vi "StopEqualization.vi"(8 "error in (no error)":errorcluster, 11 "reference in":refnum<class "niMmWave_Transceiver.lvclass">) -> (0 "error out":errorcluster, 3 "reference out":refnum<class "niMmWave_Transceiver.lvclass">)   [LabVIEW 2019, in "niMmWave_Transceiver.lvclass"]
doc: "Stops calibration procedure"
uses:
  niMmWave_Transceiver.lvclass
  C:/Barkhausen mmWave radar/Development/LV/Barkhausen mmWave hardware control/Host/SubVIs/mmWave instrument_class/mmWave instrument.lvclass
  mmWave instrument_class/Instrument state.ctl
  Low-level/TypeDefs/TX FPGA Reference.ctl
  <vilib>/Utility/error.llb/Error Cluster From Error Code.vi
  <vilib>/rvi/errors/niLvFpgaAdjustHostInterfaceError.vi
  <vilib>/rvi/interface/nirviReadWriteControl/nirviReadWriteControl.xnode
  NiFpgaLv.dll
  <vilib>/rvi/interface/Simulation/niFpgaSimulationCallBeginRW.vi
  mmWave instrument_class/mmWave instrument.lvclass
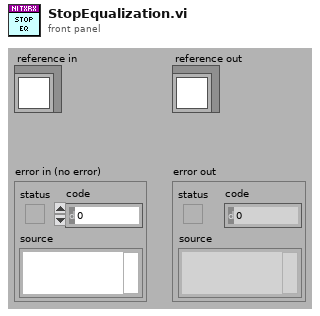
[diagram p1: front panel]
types:
  T1 = typedef "mmWave instrument.lvclass/Instrument state.ctl" = enum16{"Off", "Initialization", "Configuration", "Running", "Calibration"}
  T2 = enum16{"Pass Through", "Tone", "Pulse", "Disable"}
  T3 = typedef "TX FPGA Reference.ctl" = refnum<k20>
  T4 = typedef "niMmWave_Transceiver.lvclass/ObjectAttributesRef.ctl" = refnum<data-value>
  T5 = typedef "niMmWave_Transceiver.lvclass/ObjectAttributes.ctl" = cluster{"session":T6[], "HW.RX resources":T20, "RF config":T21, "RX trigger options":T22, "TX trigger options":T22, "RX samples":i32, "Downloaded Bursts":map{string, T25}, "TX Fs":dbl, "RX Fs":dbl, "burst sequence":string[]}
  T6 = typedef "Session.ctl" = cluster{"3620 session":refnum<queue>, "tx baseband session":T7, "rx baseband session":T15, "tx gain (dB)":dbl, "rx gain (dB)":dbl, "hardware configuration":T16, "gain ranging":T18[], "pxi trigger bus information":T19}
  T7 = typedef "Tx Baseband Session.ctl" = cluster{"3610 session":T8, "7902 reference":T14}
  T8 = typedef "ni3610_and_ni3630_Driver_Lib.lvlib/Main Settings.ctl" = cluster{"VISA resource name":refnum<visa-resource-name>, "Address Space":T9, "window_offset":u32, "register_addresses":T10, "required_MM_fpga_version":cluster{"signature":u32, "hardware":u32, "current revision":u32, "oldest revision":u32}, "CPLD Oldest Compat Version ":cluster{"hardware":u32, "CPLD firmware":u32}, "MM_FPGA_image_location":string, "is_init":bool, "card_type":T11, "DacLmkConfigFileName":string, "AdcLmkConfigFileName":string, "AdcConfigFileName":string, "DacConfigFileName_RevA":string, "DacConfigFileName_RevB":string, "Mulde hardware revision":u8, "bypass DAC PLL\n":bool, "IQ Card Revision":T12, "board capability":T13}
  T9 = typedef "VISA Register Access Address Space.ctl" = u16
  T10 = typedef "ni3610_and_ni3630_Driver_Lib.lvlib/Register Adresses.ctl" = cluster{"MM based Registers":cluster{"Revision":u32, "OldestCompatRev":u32, "signature":u32, "scratch":u32, "LedControl":u32, "BoardHwRev":u32, "BoardControl":u32, "ThermalStatus":u32, "BasebandStatus":u32, "BasebandControl":u32, "BasebandAuxSetup":u32, "BasebandAuxStatus":u32, "LmkSyncOutSetup":u32, " AdcSyncOutSetup":u32, " InjSyncOutSetup":u32, " PxiTrig0OutSetup":u32, " PxiTrig1OutSetup":u32, " PxiTrig2OutSetup":u32, " PxiTrig3OutSetup":u32, " PxiTrig4OutSetup":u32, " PxiTrig5OutSetup":u32, " PxiTrig6OutSetup":u32, " PxiTrig7OutSetup":u32}, "CPLD based Registers":cluster{"SlaveSignature":u32, "SlaveRevision":u32, "SlaveOldestCompatRev":u32, "SlaveScratch":u32, "SlaveSetup":u32, "SlaveStatus":u32, "IDacReg_offset":u32, "LMKRegGrp0_offset":u32, "QDacReg_offset":u32, "BrdTempSensorVal":u32, "TempSensorPowerDown":u32, "GPIOReg_offset":u32, "IAdcReg_offset":u32, "QAdcReg_offset":u32, "LMKRegGrp1_offset":u32, "QadcTempSensorVal":u32, "IadcTempSensorVal":u32, "RevisionReg":u32, "VcxoReg":u32, "CpldStatusReg":u32, "PowerReg":u32, "VBiasEnReg":u32, "ExtRefOeReg":u32, "QdacCtrlReg":u32, "QdacStatusReg":u32, "IdacCtrlReg":u32, "IdacStatusReg":u32, "QdacJtagIn":u32, "QdacJtagOut":u32, "IdacJtagIn":u32, "IdacJtagOut":u32, "IqDcSetupReg":u32, "QadcStatusReg":u32, "IadcStatusReg":u32, "BrdSetupReg":u32, "IqDcRevisionReg":u32, "PllStatusReg":u32, "EndpointScratchReg":u32, "AdcSyncCfgReg":u32, "IqCardOpampReg":u32}, "CPLD Register Offset":u32, "MM  Register Offset":u32, " PxiTrig0OutSetup":u32}
  T11 = typedef "ni3610_and_ni3630_Driver_Lib.lvlib/Base Card Type.ctl" = enum16{"unspecified", "ADC", "DAC"}
  T12 = typedef "ni3610_and_ni3630_Driver_Lib.lvlib/IQ Card Revision.ctl" = enum16{"RevA", "RevB", "RevC", "RevD"}
  T13 = typedef "ni3610_and_ni3630_Driver_Lib.lvlib/Board Capability.ctl" = cluster{"baseband sync":enum16{"no baseband sync", "baseband sync"}}
  T14 = typedef "Blank FPGA Reference.ctl" = refnum<k20>
  T15 = typedef "Rx Baseband Session.ctl" = cluster{"3630 session":T8, "7902 reference":T14}
  T16 = typedef "Hardware Configuration.ctl" = cluster{"direction":T17, "baseband only":bool}
  T17 = typedef "Direction.ctl" = enum16{"Transceiver", "Receiver", "Transmitter"}
  T18 = typedef "Gain Ranging.ctl" = cluster{"gain ranging active scope":string, "gain ranging stream session":refnum<k20>}
  T19 = typedef "PXI Trigger Bus Info.ctl" = cluster{"chassis resource name":refnum<visa-resource-name>, "7902R (TX)":i16, "3610 (TX)":i16, "3620 (IF)":i16, "3630 (RX)":i16, "7902R (RX)":i16}
  T20 = typedef "mmWave HW Control.lvlib/HW TXRX resources cluster.ctl" = cluster{"TX_DAC":refnum<visa-resource-name>, "TX_FPGA":tag, "IF":tag, "RX_ADC":refnum<visa-resource-name>, "RX_FPGA":tag}
  T21 = typedef "mmWave HW Control.lvlib/HW TXRX RF config cluster.ctl" = cluster{"TX.Frequency":dbl, "TX.Gain":dbl, "TX.mmWave adapter":string, "RX.Frequency":dbl, "RX.Gain":dbl, "RX.mmWave adapter":string}
  T22 = typedef "TX trigger config.ctl" = cluster{"delay":dbl, "trig source":T23, "PXI src":i32, "export":T24, "PXI dest":i32}
  T23 = typedef "FPGA Utility.lvlib/FPGA driver trigger source.ctl" = enum16{"Use Tclk", "PXI_Trig", "Aurora RX trig"}
  T24 = typedef "FPGA Utility.lvlib/FPGA driver trigger destination.ctl" = enum16{"None", "Source trig", "Synced trig", "Delayed sync"}
  T25 = typedef "niMmWave_Transceiver.lvclass/BurstInfo.ctl" = cluster{"starting addr":u32, "end addr":u32}
  T26 = cluster{"generation select":enum16{"Pass Through", "Tone", "Pulse", "Disable"}, "tone parameters":cluster{"frequency":fxp<+/-,48,0>, "gain":fxp<+/-,18,1>}, "pulse parameters":cluster{"frequency":u32, "gain":fxp<+/-,18,1>, "width":u8}}
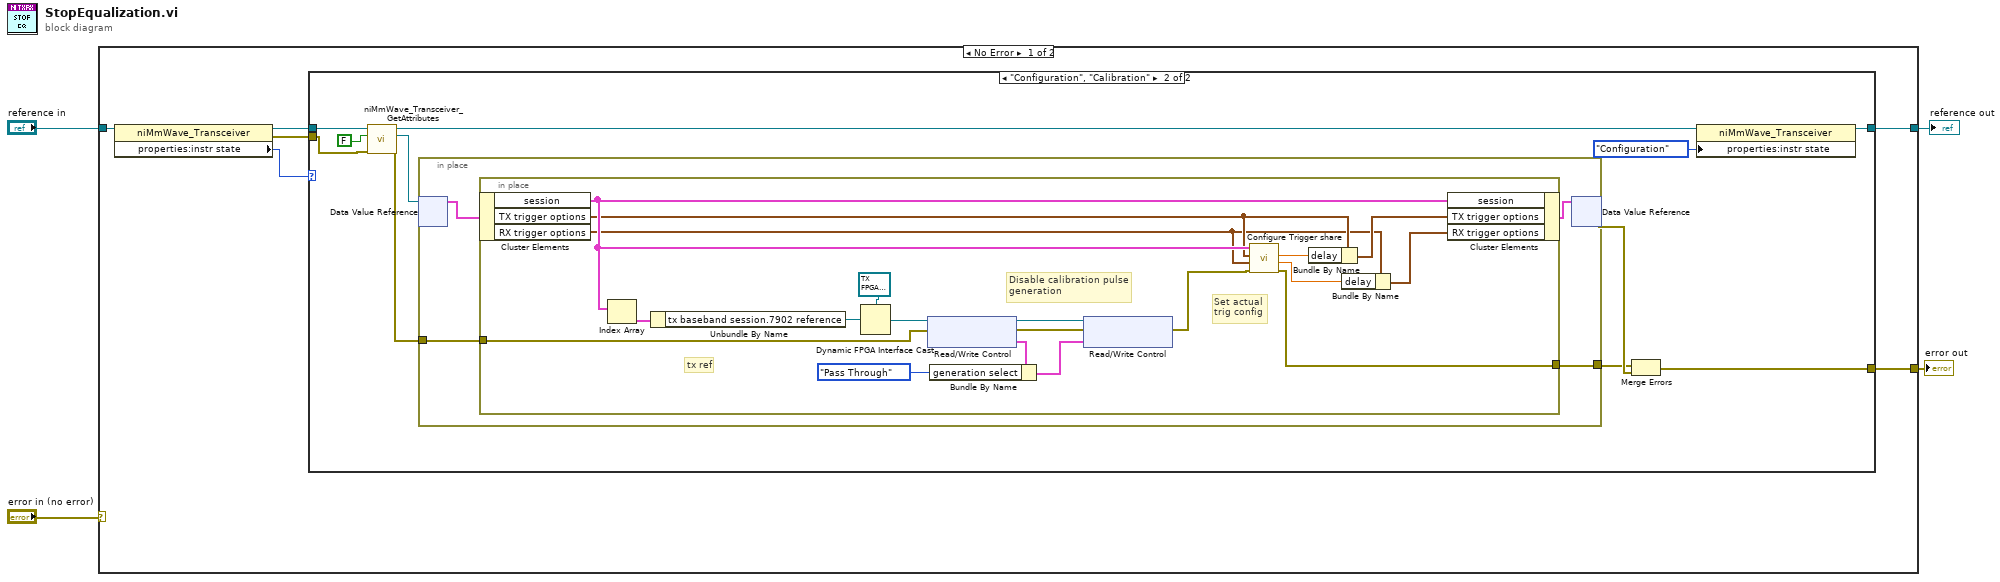
[diagram p0: block diagram]
diagram:
  n1 = case shown="No Error" "error in (no error)" {
    selector: "error in (no error)" -> [_ w48]
    tunnel: [w10 w48] -> w3
    tunnel: [w8 w47] -> w1
    tunnel: "reference in" -> [w9 w47]
    frame No Error {
      n2 = property class="niMmWave_Transceiver"(reference=w9) -> (reference out=w7:refnum<class "niMmWave_Transceiver.lvclass">, error out=w6:errorcluster, "properties:instr state"=w5:T1)  [unwired: 1 in]
      n3 = case shown="\"Configuration\", \"Calibration\"" w5 {
        tunnel: [w11 w23] -> w10
        tunnel: [w12 w14] -> w8
        tunnel: w7 -> [w12 w16]
        tunnel: w6 -> [w11 w15]
        frame "Off", Default {
        }
        frame "Configuration", "Calibration" {
          n4 = call "niMmWave_Transceiver_GetAttributes.vi"("error in (no error)"=w15, "return data? (T)"=FALSE, "reference in"=w16) -> ("error out"=w19:errorcluster, "attributes ref"=w17:T4, "reference out"=w18:refnum<class "niMmWave_Transceiver.lvclass">)  [unwired: 5 in, 1 out]
          n5 = in-place {
            in-place-border: w19 -> [w25]
            in-place-border: [w24] -> w21
            n6 = in-place-dvr #1(w17) -> (w26:T5)  [unwired: 1 out]
            n7 = in-place {
              in-place-border: w25 -> [w31]
              in-place-border: [w30] -> w24
              # "Set actual\ntrig config"
              # "Disable calibration pulse\ngeneration"
              # "tx ref"
              n8 = in-place-cluster #2(w26) -> ("session"=w34:T6[], "TX trigger options"=w29:T22, "RX trigger options"=w28:T22)
              n9 = Index Array(array=w34) -> (element=w39:T6)  [unwired: 1 in]
              n10 = Unbundle By Name(w39) -> ("tx baseband session.7902 reference"=w38:T14)
              n11 = Dynamic FPGA Interface Cast(Session In=T3 refnum ("Refnum in"), Type=w38) -> (Session Out=w46:T3)
              n12 = xnode "Read/Write Control"("FPGA VI Reference In"=w46, "error in"=w31) -> ("FPGA VI Reference Out"=w45:T3, "error out"=w44:errorcluster, "cal.generation"=w42:T26)
              n13 = Bundle By Name(cluster=w42, "generation select"=T2."Pass Through") -> (w40:T26)
              n14 = xnode "Read/Write Control"("FPGA VI Reference In"=w45, "error in"=w44, "cal.generation"=w40) -> ("error out"=w35:errorcluster)  [unwired: 1 out]
              n15 = call "Configure Trigger share.vi"("error in"=w35, "RX trigger options"=w28, "TX trigger options"=w29, "session in"=w34) -> ("error out"=w30:errorcluster, "actual rx delay"=w36:dbl, "actual tx delay"=w37:dbl)  [unwired: 4 in, 1 out]
              n16 = Bundle By Name(cluster=w29, "delay"=w37) -> (w33:T22)
              n17 = Bundle By Name(cluster=w28, "delay"=w36) -> (w32:T22)
              n18 = in-place-cluster #2("session"=w34, "TX trigger options"=w33, "RX trigger options"=w32) -> (w27:T5)
            }
            n19 = in-place-dvr #1(w27) -> (w22:errorcluster)  [unwired: 1 out]
          }
          n20 = Merge Errors(w21, w22) -> (w23:errorcluster)
          n21 = property class="niMmWave_Transceiver"(reference=w18, "properties:instr state"=Instrument_state."Configuration" ("instr state")) -> (reference out=w14:refnum<class "niMmWave_Transceiver.lvclass">)  [unwired: 1 in, 1 out]
        }
      }
    }
    frame Error {
    }
  }
  "error out" <- w3
  "reference out" <- w1
